vi "select greater.vi"(1 "Array 1 in":dbl[](array[numeric]), 6 "Array 2 in":dbl[](array[numeric])) -> (21 "Array of higher vals":dbl[](array[numeric]), 26 "Array of lower vals":dbl[](array[numeric]))   [LabVIEW 2018]
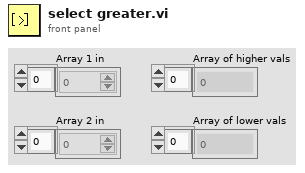
[diagram p1: front panel]
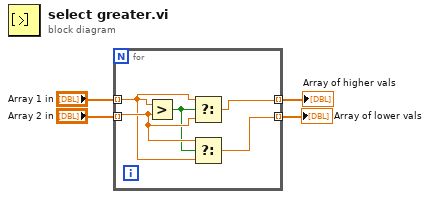
[diagram p0: block diagram]
diagram:
  n1 = for {
    tunnel: "Array 1 in" -> [w7] mode=indexing
    tunnel: "Array 2 in" -> [w8] mode=indexing
    tunnel: [w9] -> w2 mode=indexing
    tunnel: [w5] -> w1 mode=indexing
    n2 = Greater?(x=w7, y=w8) -> (0:w6:bool)
    n3 = Select(t=w7, s=w6, f=w8) -> (s? t:f=w9:dbl)
    n4 = Select(t=w8, s=w6, f=w7) -> (s? t:f=w5:dbl)
  }
  "Array of lower vals" <- w1
  "Array of higher vals" <- w2
